vi "Publisher.vi"() -> ()   [LabVIEW 2014]
uses:
  ROS-for-LabVIEW-Software/MoreExample/ctl/pose.ctl
  <vilib>/Tufts CEEO ROS for LabVIEW Software/ROS/Code/Console/Servers/ServerSubs/TopicDef.ctl
  <vilib>/Tufts CEEO ROS for LabVIEW Software/ROS/Code/SubVIs/_ROSDirection.ctl
  ctl/Point.ctl
  ctl/RPY.ctl
panel:
  out "error out 2":errorcluster
  out "输出簇":T1
  out "msg out":string
  out "Quaternion":cluster{"x":dbl, "y":dbl, "z":dbl, "w":dbl}
  out "error out":errorcluster
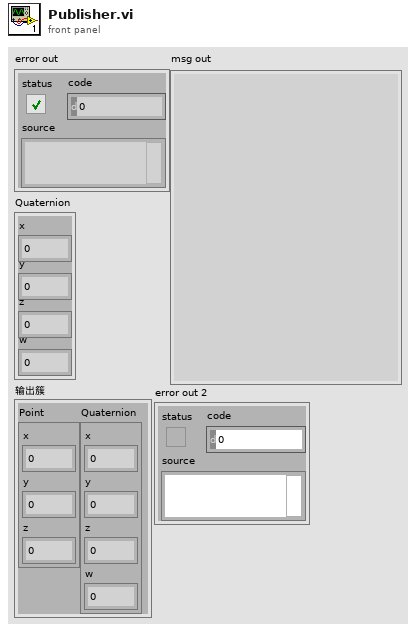
[diagram p1: front panel]
types:
  T1 = typedef "pose.ctl" = cluster{"Point":cluster{"x":dbl, "y":dbl, "z":dbl}, "Quaternion":cluster{"x":dbl, "y":dbl, "z":dbl, "w":dbl}}
  T2 = typedef "TopicDef.ctl" = cluster{"Topic":string, "Type":string, "Action":T3, "Update (ms)":u16, "queue size":u16}
  T3 = typedef "_ROSDirection.ctl" = enum16{"Node", "Publisher", "Subscriber", "ServiceClient", "ServiceProvider"}
  T4 = typedef "_ROSControl.ctl" = cluster{"topic port":u16, "Node":string, "topic":string, "type":string, "node port":u16, "error ":errorcluster, "Direction":T3, "Update (ms)":u16, "FIFO size":u16}
  T5 = typedef "RPY.ctl" = cluster{"Roll (y)":dbl, "Pitch (x)":dbl, "Yaw (z)":dbl}
  T6 = typedef "Point.ctl" = cluster{"x":dbl, "y":dbl, "z":dbl}
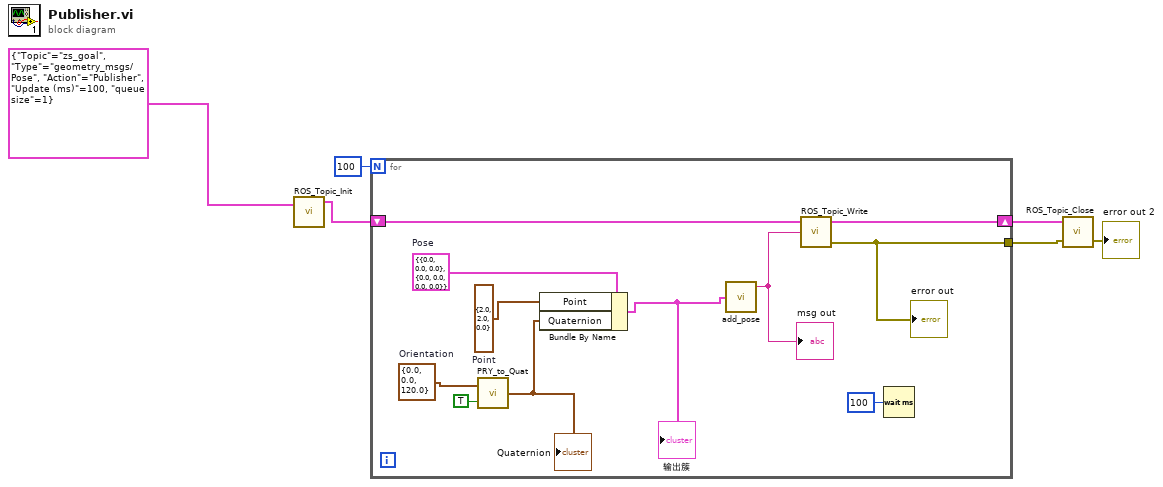
[diagram p0: block diagram]
diagram:
  n1 = call <vilib>:"ROS_Topic_Init.vi"("Definitions"=T2 {"Topic"="zs_goal", "Type"="geometry_msgs/Pose", "Action"=enum."Publisher", "Update (ms)"=100, "queue size"=1}) -> ("ROS out"=w3:T4)  [unwired: 2 in, 1 out]
  n2 = for {
    N: 100 -> [_]
    tunnel: [w17] -> w6
    shift-right: [w16] -> w5
    shift-left: w3 -> [w15]
    w13 = T5 {"Roll (y)"=0.0, "Pitch (x)"=0.0, "Yaw (z)"=120.0}  # Orientation
    w11 = T6 {"x"=2.0, "y"=2.0, "z"=0.0}  # Point
    w12 = T1 {"Point"={"x"=0.0, "y"=0.0, "z"=0.0}, "Quaternion"={"x"=0.0, "y"=0.0, "z"=0.0, "w"=0.0}}  # Pose
    n3 = call <vilib>:"PRY_to_Quat.vi"("From Degrees? (T)"=TRUE, "Orientation"=w13) -> ("Quaternion"=w10:cluster{"x":dbl, "y":dbl, "z":dbl, "w":dbl})
    "Quaternion" <- w10
    n4 = Bundle By Name(cluster=w12, "Point"=w11, "Quaternion"=w10) -> (w8:T1)
    "输出簇" <- w8
    n5 = call <vilib>:"add_pose.vi"("Pose"=w8) -> ("msg out"=w9:string)  [unwired: 4 in]
    "msg out" <- w9
    n6 = call <vilib>:"ROS_Topic_Write.vi"("Msg in"=w9, "ROS in"=w15) -> ("error out"=w17:errorcluster, "ROS out"=w16:T4)  [unwired: 2 in]
    "error out" <- w17
    n7 = Wait (ms)(milliseconds to wait=u32 100 ("等待时间（毫秒）")) -> ()  [unwired: 1 out]
  }
  n8 = call <vilib>:"ROS_Topic_Close.vi"("error in"=w6, "ROS in"=w5) -> ("error out"=→"error out 2":errorcluster)  [unwired: 2 in]
